vi "Tek_Init.vi"(11 "VISA":refnum<visa-resource-name>) -> (0 "error out":errorcluster, 2 "replies":string[](array[string]))   [LabVIEW 2022 SP3]
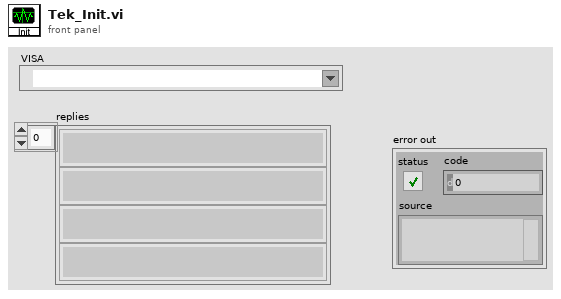
[diagram p1: front panel]
types:
  T1 = cluster{"write buffer":string, "byte count":u32}[]
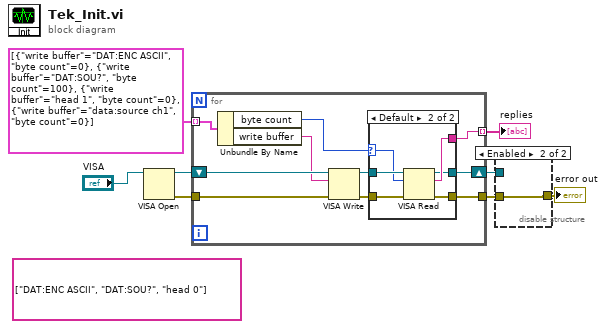
[diagram p0: block diagram]
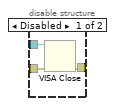
[diagram p2: hidden frame]
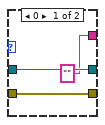
[diagram p3: hidden frame]
diagram:
  (unwired) string[] ["DAT:ENC ASCII", "DAT:SOU?", "head 0"]
  n1 = VISA Open(VISA resource name="VISA") -> (VISA resource name=w4:refnum<visa-resource-name>, error out=w7:errorcluster)  [unwired: 4 in]
  n2 = for {
    tunnel: [w16] -> w5 mode=indexing
    shift-right: [w15] -> w3
    shift-left: w4 -> [w18]
    tunnel: w7 -> [w13]
    tunnel: [w12] -> w2
    tunnel: T1 [{"write buffer"="DAT:ENC ASCII", "byte count"=0}, {"write buffer"="DAT:SOU?", "byte count"=100}, {"write buffer"="head 1", "byte count"=0}, {"write buffer"="data:source ch1", "byte count"=0}] -> [w11] mode=indexing
    n3 = Unbundle By Name(w11) -> ("byte count"=w10:u32, "write buffer"=w9:string)
    n4 = VISA Write(VISA resource name=w18, write buffer=w9, error in (no error)=w13) -> (VISA resource name out=w14:refnum<visa-resource-name>, error out=w17:errorcluster)  [unwired: 1 out]
    n5 = case shown="Default" w10 {
      selector: w10 -> [_ w22]
      tunnel: w17 -> [w20 w27]
      tunnel: ["" ("read buffer") w26] -> w16
      tunnel: [w21 w25] -> w15
      tunnel: w14 -> [w21 w24]
      tunnel: [w20 w23] -> w12
      frame 0 {
      }
      frame Default {
        n6 = VISA Read(VISA resource name=w24, byte count=w22, error in (no error)=w27) -> (VISA resource name out=w25:refnum<visa-resource-name>, read buffer=w26:string, error out=w23:errorcluster)  [unwired: 1 out]
      }
    }
  }
  "replies" <- w5
  n7 = disable-structure shown="Enabled" {
    disable-tunnel: w3 -> [w30 _]
    disable-tunnel: w2 -> [w29 w31]
    disable-tunnel: [w28 w31] -> w1
    frame Disabled {
      n8 = VISA Close(VISA resource name=w30, error in (no error)=w29) -> (error out=w28:errorcluster)
    }
    frame Enabled {
    }
  }
  "error out" <- w1
